vi "Implement IIR Direct Filter for N Chan (CDB).vi"(7 "reset Filters":bool[](array[boolean]), 8 "error in (no error)":errorcluster, 9 "Forward Coefficients":dbl[](array[numeric]) format="%0.2f", 10 "Reverse Coefficients":dbl[](array[numeric]) format="%0.2f", 11 "arrWaveforms In":waveform(cdb)[](array[waveform])) -> (0 "error out":errorcluster, 3 "arrWaveforms Out":waveform(cdb)[](array[waveform]))   [LabVIEW 2020, in "NI_MAPro.lvlib"]
uses:
  NI_MAPro.lvlib
  NI_MABase.lvlib
  NI_AALBase.lvlib
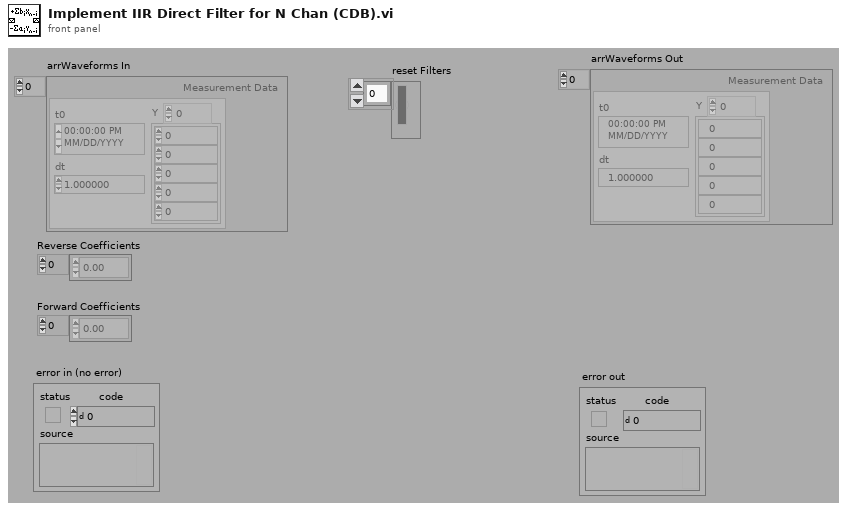
[diagram p1: front panel]
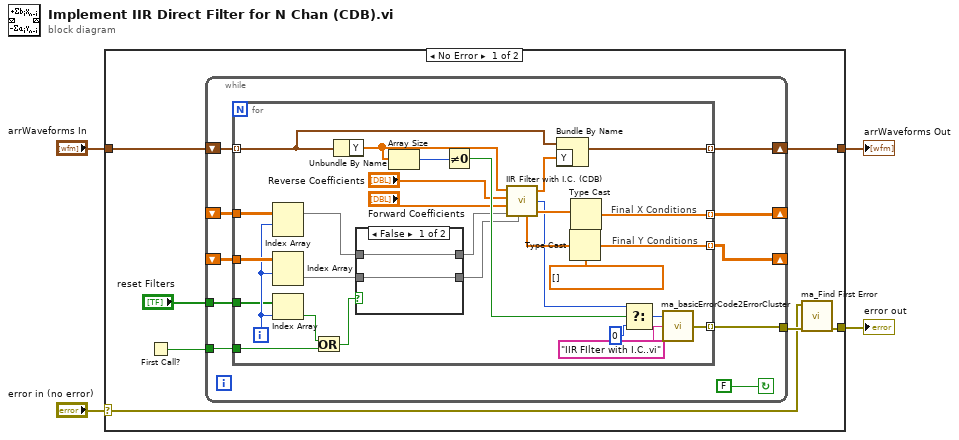
[diagram p0: block diagram]
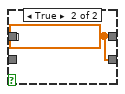
[diagram p2: hidden frame]
diagram:
  n1 = case shown="No Error" "error in (no error)" {
    selector: "error in (no error)" -> [w7 w55]
    tunnel: [w10 w55] -> w4
    tunnel: "arrWaveforms In" -> [w9 w54]
    tunnel: [w8 w54] -> w1
    frame No Error {
      n2 = First Call?() -> (First Call?: T/F=w5:bool)
      n3 = while {
        tunnel: "reset Filters" -> [w14]
        tunnel: [w13] -> w11
        shift-left: w9 -> [w16]
        shift-right: [w17] -> w8
        shift-left: _ -> [w20]
        shift-right: [w18] -> _
        shift-left: _ -> [w21]
        shift-right: [w19] -> _
        tunnel: w5 -> [w12]
        stop <- FALSE continue-if-true
        n4 = for {
          tunnel: w21 -> [w44]
          tunnel: w20 -> [w45]
          tunnel: [w49] -> w19 mode=indexing
          tunnel: [w48] -> w18 mode=indexing
          tunnel: [w46] -> w17 mode=indexing
          tunnel: w16 -> [w36] mode=indexing
          tunnel: [w31] -> w13 mode=indexing
          tunnel: w14 -> [w32]
          tunnel: w12 -> [w22]
          i -> [w33]
          w47 = cdb[] [] ("type for the shift register")
          # "Final Y Conditions"
          # "Final X Conditions"
          n5 = Index Array(array=w44, index (row)=w33) -> (element=w38:cdb[])  [unwired: 1 in]
          n6 = Index Array(array=w45, index (row)=w33) -> (element=w34:cdb[])  [unwired: 1 in]
          n7 = Index Array(array=w32, index=w33) -> (element=w24:bool)
          n8 = Or(x=w24, y=w22) -> (x .or. y?=w23:bool)
          n9 = Unbundle By Name(w36) -> ("Y"=w25:cdb[])
          n10 = case shown="False" w23 {
            tunnel: w34 -> [w52 _]
            tunnel: [w52 w53] -> w39
            tunnel: w38 -> [w51 _]
            tunnel: [w51 w53] -> w37
            frame False {
            }
            frame True {
              w53 = cdb[] [] ("type for the shift register")
            }
          }
          n11 = Array Size(array=w25) -> (size(s)=w26:i32)
          n12 = Not Equal To 0?(x=w26) -> (x != 0?=w50:bool)
          n13 = call "IIR Filter with I.C. (CDB).vi"("Initial Y Conditions"=w39, "Initial X Conditions"=w37, "Forward Coefficients"="Forward Coefficients", "Reverse Coefficients"="Reverse Coefficients", "X"=w25) -> ("Final X Conditions"=w43:cdb[], "Final Y Conditions"=w42:cdb[], "error"=w27:i32, "Filtered X"=w35:cdb[])  [unwired: 2 in]
          n14 = Bundle By Name(cluster=w36, "Y"=w35) -> (w46:waveform(cdb))
          n15 = Type Cast(type=w47, x=w42) -> (*(type *) &x=w48:cdb[])
          n16 = Type Cast(type=w47, x=w43) -> (*(type *) &x=w49:cdb[])
          n17 = Select(t=w27, s=w50, f=0) -> (s? t:f=w28:i32)
          n18 = call "ma_basicErrorCode2ErrorCluster.vi"("subVI name"="IIR FIlter with I.C..vi", "Error Code"=w28) -> ("error out"=w31:errorcluster)  [unwired: 1 in]
        }
      }
      n19 = call "ma_Find First Error.vi"("error array in"=w11, "error in 1 (no error)"=w7) -> ("error out"=w10:errorcluster)  [unwired: 5 in]
    }
    frame Error {
    }
  }
  "error out" <- w4
  "arrWaveforms Out" <- w1
